vi "בדיקת זמן מיתוג הממסר 5.vi"(7 "resultUserPrompt":bool, 8 "error":errorcluster, 10 "lines":tag="PXI1Slot8/port0/line1", 11 "Path for Log":path) -> (0 "error out":errorcluster, 1 "בטוח כן/לא":bool, 2 "בדיקת זמן מיתוג הממסר":dbl)   [LabVIEW 2015]
uses:
  <instrlib>/niDMM/nidmm.llb/niDMM Function.ctl
  <instrlib>/niDMM/nidmm.llb/niDMM Resolution in Digits.ctl
  <vilib>/DAQmx/write.llb/DAQmx Write (Digital Bool 1Line 1Point).vi
  <instrlib>/niDMM/nidmm.llb/niDMM Configure Measurement Digits.vi
  <vilib>/DAQmx/create/channels.llb/DAQmx Create Channel (DO-Digital Output).vi
  <vilib>/DAQmx/miscellaneous.llb/DAQmx Fill In Error Info.vi
panel:
  in  "התחל":bool
  # "Right-Click to\nexplain error"
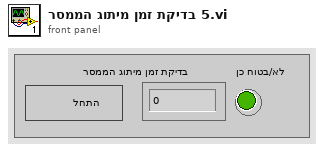
[diagram p1: front panel]
types:
  T1 = enum32{"Invalid", "Standard", "Closed", "Hidden", "Minimized", "Maximized"}
  T2 = typedef "niDMM Function.ctl" = enum16{"DC Volts", "AC Volts", "DC Current", "AC Current", "2-wire Resistance", "4-wire Resistance", "Diode", "Frequency", "Period", "AC Volts DC Coupled", "Capacitance", "Inductance", "Temperature"}
  T3 = typedef "niDMM Resolution in Digits.ctl" = dbl
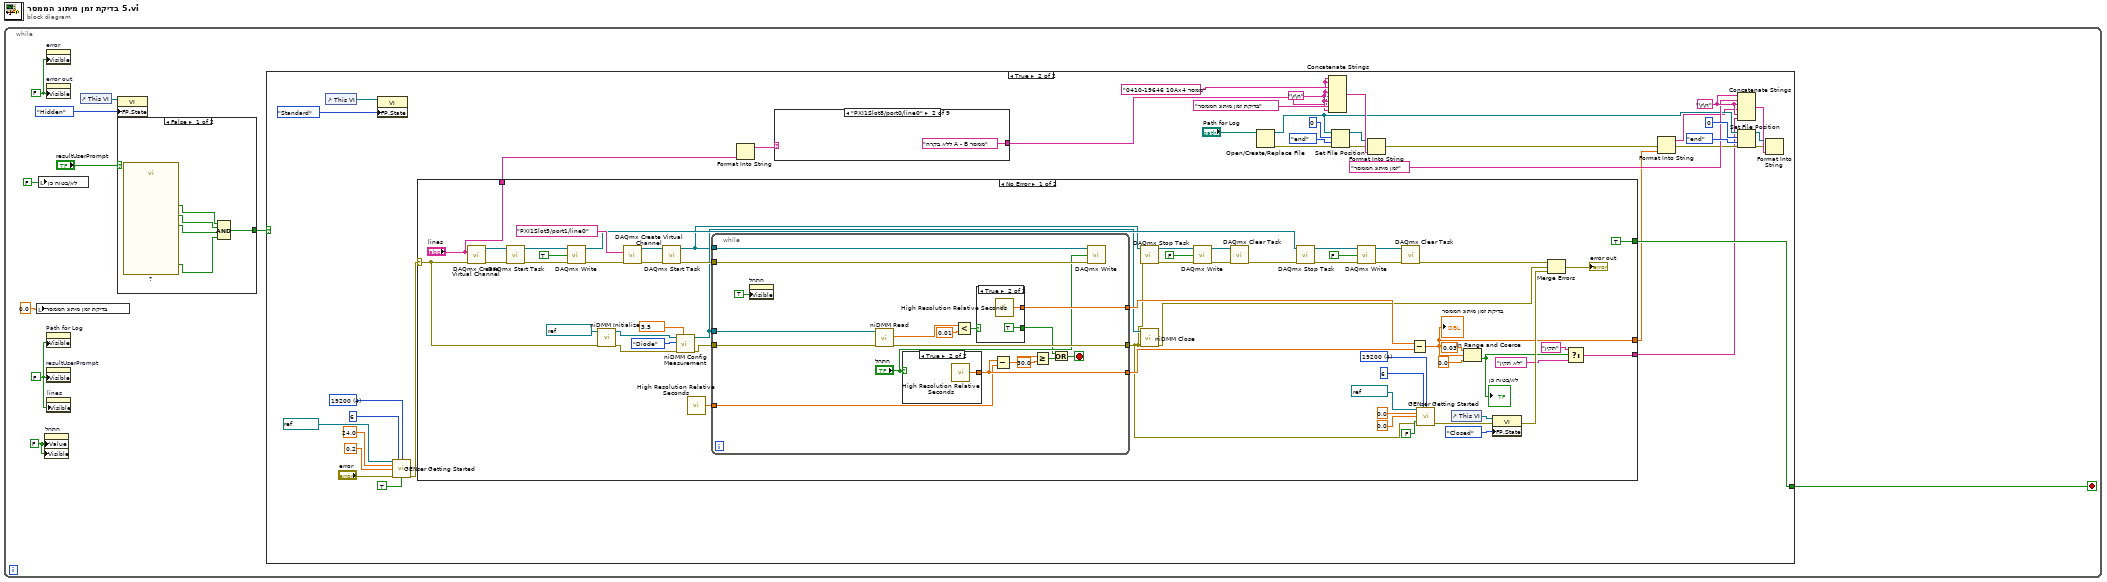
[diagram p0: block diagram]
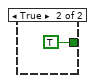
[diagram p2: hidden frame]
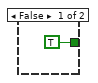
[diagram p3: hidden frame]
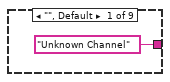
[diagram p4: hidden frame]
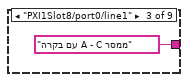
[diagram p5: hidden frame]
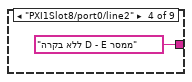
[diagram p6: hidden frame]
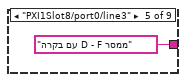
[diagram p7: hidden frame]
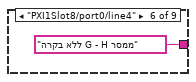
[diagram p8: hidden frame]
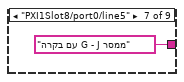
[diagram p9: hidden frame]
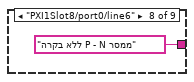
[diagram p10: hidden frame]
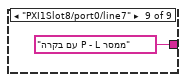
[diagram p11: hidden frame]
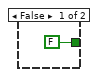
[diagram p12: hidden frame]
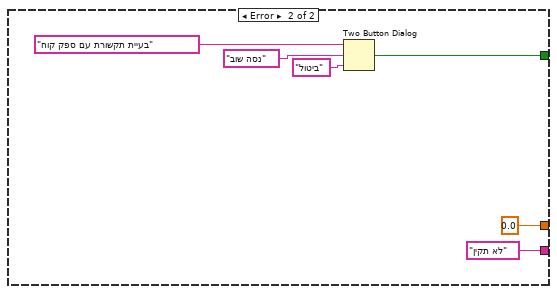
[diagram p14: hidden frame]
diagram:
  n1 = while {
    stop <- w2 stop-if-true
    w1 = FALSE ("data")
    w3 = FALSE ("Visible")
    w10 = FALSE ("Visible")
    n2 = local write "בדיקת זמן מיתוג הממסר"(0.0 ("בדיקת זמן מיתוג הממסר")) -> ()
    n3 = local write "בטוח כן/לא"(FALSE ("בטוח כן/לא")) -> ()
    n4 = property on="התחל" class="Bool (strict)"("Value"=w1, "Visible"=w1) -> ()  [unwired: 2 in, 2 out]
    n5 = property on="error" class="Clust (strict)"("Visible"=w10) -> ()  [unwired: 2 in, 2 out]
    n6 = property on="error out" class="Clust (strict)"("Visible"=w10) -> ()  [unwired: 2 in, 2 out]
    n7 = property on="Path for Log" class="Path"("Visible"=w3) -> ()  [unwired: 2 in, 2 out]
    n8 = property on="resultUserPrompt" class="Bool (strict)"("Visible"=w3) -> ()  [unwired: 2 in, 2 out]
    n9 = property on="lines" class="DAQmxName"("Visible"=w3) -> ()  [unwired: 2 in, 2 out]
    n10 = control-ref of="This VI"() -> (w9:refnum<vi>)
    n11 = property class="VI"(reference=w9, "FP.State"=T1."Hidden" ("Front Panel Window:State")) -> ()  [unwired: 1 in, 2 out]
    n12 = case shown="False" "resultUserPrompt" {
      tunnel: [w15 TRUE] -> w7
      frame False {
        n13 = call "?"() -> ("הדקי הרב מודד"=w11:bool, "M מגע שלילי"=w12:bool, "K מגע חיובי"=w13:bool, "OK"=w14:bool)  [unwired: 15 in, 1 out]
        n14 = Compound Arithmetic op=AND(w14, w13, w12, w11) -> (w15:bool)
      }
      frame True {
      }
    }
    n15 = case shown="True" w7 {
      tunnel: [TRUE ("T button?") w47] -> w2
      frame False {
      }
      frame True {
        w32 = "\r\n"
        w19 = "\r\n"
        w50 = u16 4 items=["1200", "2400", "4800", "9600", "19200"] ("BAUD")
        n16 = control-ref of="This VI"() -> (w46:refnum<vi>)
        n17 = property class="VI"(reference=w46, "FP.State"=T1."Standard" ("Front Panel Window:State")) -> ()  [unwired: 1 in, 2 out]
        n18 = call "GENser Getting Started.vi"("VISA"=refnum<visa-resource-name> "COM6", "GEN Addr"=i16 6, "BAUD"=w50, "Voltage Limit"=24.0, "Current Limit"=0.2, "error"="error", "Output On (T)"=TRUE) -> ("error out"=w52:errorcluster)  [unwired: 5 in, 3 out]
        n19 = case shown="No Error" w52 {
          selector: w52 -> [w67 _]
          tunnel: [TRUE ("T button?") w145] -> w47
          tunnel: [w98 0.0] -> w24
          tunnel: [w94 "לא תקין"] -> w23
          tunnel: ["lines" _] -> w21
          frame No Error {
            w71 = T3 3.5 items=["3 1/2"=3.5, "4 1/2"=4.5, "5 1/2"=5.5, "6 1/2"=6.5, "7 1/2"=7.5] ("Resolution in Digits")
            w114 = u16 4 items=["1200", "2400", "4800", "9600", "19200"] ("BAUD")
            n20 = call-poly <vilib>:"DAQmx Create Virtual Channel.vi"("lines"="lines", "error in"=w67) -> ("task out"=w87:refnum<k21>, "error out"=w86:errorcluster)  [unwired: 12 in]
            n21 = call <vilib>:"DAQmx Start Task.vi"("task/channels in"=w87, "error in"=w86) -> ("task out"=w84:refnum<k21>, "error out"=w85:errorcluster)  [unwired: 12 in]
            n22 = call-poly <vilib>:"DAQmx Write.vi"("task/channels in"=w84, "data"=TRUE, "error in"=w85) -> ("task out"=w75:refnum<k21>, "error out"=w73:errorcluster)  [unwired: 10 in, 1 out]
            n23 = call <instrlib>:"niDMM Initialize.vi"("error in (no error)"=w67, "Instrument Descriptor"=refnum<k15> "PXI1Slot9") -> ("error out"=w69:errorcluster, "instrument handle out"=w70:refnum<k15>)  [unwired: 8 in]
            n24 = call-poly <vilib>:"DAQmx Create Virtual Channel.vi"("lines"=tag "PXI1Slot5/port1/line0", "error in"=w73) -> ("task out"=w91:refnum<k21>, "error out"=w92:errorcluster)  [unwired: 12 in]
            n25 = call <vilib>:"DAQmx Start Task.vi"("task/channels in"=w91, "error in"=w92) -> ("task out"=w65:refnum<k21>, "error out"=w89:errorcluster)  [unwired: 12 in]
            n26 = call-poly <instrlib>:"niDMM Config Measurement.vi"("Resolution in Digits"=w71, "error in (no error)"=w69, "Function"=niDMM_Function."Diode", "instrument handle"=w70) -> ("error out"=w68:errorcluster, "instrument handle out"=w66:refnum<k15>)  [unwired: 6 in]
            n27 = call <vilib>:"High Resolution Relative Seconds.vi"() -> ("relative seconds"=w88:dbl)
            n28 = while {
              tunnel: [w131] -> w104
              tunnel: [w138] -> w105
              tunnel: [w133] -> w64
              tunnel: w65 -> [w137]
              tunnel: w89 -> [w136]
              tunnel: w88 -> [w130]
              tunnel: w66 -> [w123]
              tunnel: w68 -> [w122]
              stop <- w127 stop-if-true
              n29 = property on="התחל" class="Bool (strict)"("Visible"=TRUE ("data")) -> ()  [unwired: 2 in, 2 out]
              n30 = call <instrlib>:"niDMM Read.vi"("error in (no error)"=w122, "instrument handle"=w123) -> ("error out"=w133:errorcluster, "Measurement"=w135:dbl)  [unwired: 7 in, 1 out]
              n31 = case shown="True" "התחל" {
                tunnel: [_ w142] -> w131
                frame False {
                }
                frame True {
                  n32 = call <vilib>:"High Resolution Relative Seconds.vi"() -> ("relative seconds"=w142:dbl)
                }
              }
              n33 = Less?(x=w135, y=0.01) -> (x < y?=w124:bool)
              n34 = case shown="True" w124 {
                tunnel: [_ w141] -> w138
                tunnel: [FALSE TRUE] -> w126
                frame False {
                }
                frame True {
                  n35 = call <vilib>:"High Resolution Relative Seconds.vi"() -> ("relative seconds"=w141:dbl)
                }
              }
              n36 = Subtract(x=w131, y=w130) -> (x-y=w129:dbl)
              n37 = Greater Or Equal?(x=w129, y=30.0) -> (x >= y?=w125:bool)
              n38 = Or(x=w126, y=w125) -> (x .or. y?=w127:bool)
              n39 = call-poly <vilib>:"DAQmx Write.vi"("task/channels in"=w137, "data"="התחל", "error in"=w136) -> ()  [unwired: 10 in, 3 out]
            }
            n40 = call <vilib>:"DAQmx Stop Task.vi"("task/channels in"=w65, "error in"=w64) -> ("task out"=w110:refnum<k21>, "error out"=w109:errorcluster)  [unwired: 12 in]
            n41 = call <instrlib>:"niDMM Close.vi"("error in (no error)"=w64, "instrument handle"=w66) -> ("error out"=w102:errorcluster)  [unwired: 9 in]
            n42 = call-poly <vilib>:"DAQmx Write.vi"("task/channels in"=w110, "data"=FALSE, "error in"=w109) -> ("task out"=w107:refnum<k21>, "error out"=w108:errorcluster)  [unwired: 10 in, 1 out]
            n43 = call <vilib>:"DAQmx Clear Task.vi"("task in"=w107, "error in"=w108) -> ("error out"=w77:errorcluster)  [unwired: 13 in]
            n44 = call <vilib>:"DAQmx Stop Task.vi"("task/channels in"=w75, "error in"=w77) -> ("task out"=w78:refnum<k21>, "error out"=w80:errorcluster)  [unwired: 12 in]
            n45 = call-poly <vilib>:"DAQmx Write.vi"("task/channels in"=w78, "data"=FALSE, "error in"=w80) -> ("task out"=w81:refnum<k21>, "error out"=w82:errorcluster)  [unwired: 10 in, 1 out]
            n46 = call <vilib>:"DAQmx Clear Task.vi"("task in"=w81, "error in"=w82) -> ("error out"=w76:errorcluster)  [unwired: 13 in]
            n47 = Subtract(x=w105, y=w104) -> (x-y=w98:dbl)
            "בדיקת זמן מיתוג הממסר" <- w98
            n48 = call "GENser Getting Started.vi"("VISA"=refnum<visa-resource-name> "COM6", "GEN Addr"=i16 6, "BAUD"=w114, "Voltage Limit"=0.0, "Current Limit"=0.0, "error"=w64, "Output On (T)"=FALSE) -> ("error out"=w113:errorcluster)  [unwired: 5 in, 3 out]
            n49 = control-ref of="This VI"() -> (w112:refnum<vi>)
            n50 = In Range and Coerce(upper limit=0.03, x=w98, lower limit=0.0) -> (In Range?=w95:bool)  [unwired: 1 out]
            "בטוח כן/לא" <- w95
            n51 = property class="VI"(reference=w112, error in=w113, "FP.State"=T1."Closed" ("Front Panel Window:State")) -> (error out=w101:errorcluster)  [unwired: 1 out]
            n52 = Merge Errors(w76, w102, w101) -> (→"error out":errorcluster)
            n53 = Select(t="תקין", s=w95, f="לא תקין") -> (s? t:f=w94:string)
          }
          frame Error {
            n54 = Two Button Dialog(message="בעיית תקשורת עם ספק קוח", 1:"ביטול" ("F button name (\"Cancel\")"), 2:"נסה שוב" ("T button name (\"OK\")")) -> (T button?=w145:bool)
          }
        }
        n55 = Format Into String(w21) -> (resulting string=w22:string)  [unwired: 3 in, 1 out]
        n56 = case shown="\"PXI1Slot8/port0/line0\"" w22 {
          tunnel: ["Unknown Channel" "ללא בקרה A - B ממסר" "עם בקרה A - C ממסר" "ללא בקרה D - E ממסר" "עם בקרה D - F ממסר" "ללא בקרה G - H ממסר" "עם בקרה G - J ממסר" "ללא בקרה P - N ממסר" "עם בקרה P - L ממסר"] -> w18
          frame "", Default {
          }
          frame "PXI1Slot8/port0/line0" {
          }
          frame "PXI1Slot8/port0/line1" {
          }
          frame "PXI1Slot8/port0/line2" {
          }
          frame "PXI1Slot8/port0/line3" {
          }
          frame "PXI1Slot8/port0/line4" {
          }
          frame "PXI1Slot8/port0/line5" {
          }
          frame "PXI1Slot8/port0/line6" {
          }
          frame "PXI1Slot8/port0/line7" {
          }
        }
        n57 = Open/Create/Replace File(file path (use dialog)="Path for Log") -> (refnum out=w28:refnum<file>, error out=w29:errorcluster)  [unwired: 5 in, 1 out]
        n58 = Concatenate Strings(w19, w19, "0410-19646 10Ax4 ממסר", w19, w18, w19, "בדיקת זמן מיתוג הממסר", w19) -> (w41:string)
        n59 = Set File Position(offset (in bytes) (0)=i64 0, refnum=w28, from (0:start)=enum16{"start", "end", "current"}."end", error in=w29) -> (refnum out=w39:refnum<file>, error out=w38:errorcluster)
        n60 = Format Into String(initial string=w39, error in=w38, w41) -> (error out=w27:errorcluster)  [unwired: 1 in, 1 out]
        n61 = Format Into String(error in=w27, w24) -> (resulting string=w25:string, error out=w26:errorcluster)  [unwired: 2 in]
        n62 = Concatenate Strings(w32, "זמן מיתוג הממסר", w32, w25, w32, w23) -> (w37:string)
        n63 = Set File Position(offset (in bytes) (0)=i64 0, refnum=w28, from (0:start)=enum16{"start", "end", "current"}."end", error in=w26) -> (refnum out=w35:refnum<file>, error out=w36:errorcluster)
        n64 = Format Into String(initial string=w35, error in=w36, w37) -> ()  [unwired: 1 in, 2 out]
      }
    }
  }
